vi "FrequencyShiftOneTarget_04012019.vi"(11 "Tones in":T3={"Config"={"UsrCfg"={"Paths"={"CfgFile"=path "", "LogFolder"=path "", "LogFile"=path "", "NAS path"=path "", "ThreshFile"=path "", "RedunFolder"=path ""}, "SampleRate"=0.0}, "FP_User"={"#NoiseSums"=1, "Max_df"=1, "AvgAvg"=FALSE, "#Avg"=0, "AutoCenter"=FALSE, "Inclin"={"Vmin"=0.0, "Vmax"=0.0, "Angle_min"=0.0, "Angle_max"=0.0, "Offset"=0.0, "Pos_Neg"=FALSE}, "1"={"Cal_"={"Fine"=0.0, "Coarse_"=0.0}, "Beac"={"Fine"=0.0, "Coarse_"=0.0}, "Scale"={"Step4"=0.0, "Step5"=0.0, "Step6"=0.0, "Step7"=0.0}, "Offset"=0.0, "Scale_Noise"=0.0, "Scale_Step1"=0.0, "Scale_In_RT"=0.0, "ScaleMeas"=0.0, "FreqsToRemove"=[], "Width"=[0, 1633], "ScaleMeasEnum"=enum."50", "FilterEnab"=enum."Step 1"}, "2"={"Cal_"={"Fine"=0.0, "Coarse_"=0.0}, "Beac"={"Fine"=0.0, "Coarse_"=0.0}, "Scale"={"Step4"=0.0, "Step5"=0.0, "Step6"=0.0, "Step7"=0.0}, "Offset"=0.0, "Scale_Noise"=0.0, "Scale_Step1"=0.0, "Scale_In_RT"=0.0, "ScaleMeas"=0.0, "FreqsToRemove"=[], "Width"=[0, 1633], "ScaleMeasEnum"=enum."50", "FilterEnab"=enum."Step 1"}, "3"={"Cal_"={"Fine"=0.0, "Coarse_"=0.0}, "Beac"={"Fine"=0.0, "Coarse_"=0.0}, "Scale"={"Step4"=0.0, "Step5"=0.0, "Step6"=0.0, "Step7"=0.0}, "Offset"=0.0, "Scale_Noise"=0.0, "Scale_Step1"=0.0, "Scale_In_RT"=0.0, "ScaleMeas"=0.0, "FreqsToRemove"=[], "Width"=[0, 1633], "ScaleMeasEnum"=enum."50", "FilterEnab"=enum."Step 1"}, "4"={"Cal_"={"Fine"=0.0, "Coarse_"=0.0}, "Beac"={"Fine"=0.0, "Coarse_"=0.0}, "Scale"={"Step4"=0.0, "Step5"=0.0, "Step6"=0.0, "Step7"=0.0}, "Offset"=0.0, "Scale_Noise"=0.0, "Scale_Step1"=0.0, "Scale_In_RT"=0.0, "ScaleMeas"=0.0, "FreqsToRemove"=[], "Width"=[0, 1633], "ScaleMeasEnum"=enum."50", "FilterEnab"=enum."Step 1"}, "Target to Probe"=enum."4", "SNR_Thresh"=1.0, "Paths"={"CfgFile"=path "", "LogFolder"=path "", "LogFile"=path "", "NAS path"=path "", "ThreshFile"=path "", "RedunFolder"=path ""}, "Connex_Location"="", "SimulateFPGA"=FALSE, "Deadband"=0.0}}, "FPGA"={"Target"=enum."4", "Channel"=enum."4", "Ref1"=refnum, "Ref2"=refnum}, "Now"={"Target"=enum."4", "SampleRate"=0.0, "AvgFreq"=0.0, "72_Shift_"=-24999462.633451957, "84_Shift_"=-24999462.633451957, "1"={"Cal"={"Shift_"=0.0, "Peak_ToFPGA"=-24999462.633451957, "MaxValue"=0.0, "MaxIndex"=0, "Tone"={"PkLocTrak"=0.0, "PkLocDisp"=0.0, "df_"=0.0, "ZoomPwr"=[], "Phase"=0.0, "PhaseOld"=0.0, "AboveThresh?"=FALSE, "MaxI"=0.0, "MaxQ"=0.0, "median"=0.0, "ISpect"=[], "QSpect"=[], "DeltaPhase"=0.0}, "TimeDomainI"=array[12500 elements], "TimeDomainQ"=array[12500 elements], "PwrSpectrum"=[], "RunningAvgFreq"=0.0, "ISpectPos"=[], "ISpectNeg"=[], "QSpectPos"=[], "QSpectNeg"=[], "10Hz_PwrSpectr"=[], "SNR"=0.0, "AliasWarn"=FALSE, "10Hz_Peak"=[], "ISpect+-"=[], "QSpect+-"=[], "TimeStamp"=timestamp(0 s since 1904-01-01), "I_Index"=array[12500 elements], "Q_Index"=array[12500 elements], "10MHz"=FALSE}, "Beac"={"Shift_"=0.0, "Peak_ToFPGA"=-24999462.633451957, "MaxValue"=0.0, "MaxIndex"=0, "Tone"={"PkLocTrak"=0.0, "PkLocDisp"=0.0, "df_"=0.0, "ZoomPwr"=[], "Phase"=0.0, "PhaseOld"=0.0, "AboveThresh?"=FALSE, "MaxI"=0.0, "MaxQ"=0.0, "median"=0.0, "ISpect"=[], "QSpect"=[], "DeltaPhase"=0.0}, "TimeDomainI"=array[12500 elements], "TimeDomainQ"=array[12500 elements], "PwrSpectrum"=[], "RunningAvgFreq"=0.0, "ISpectPos"=[], "ISpectNeg"=[], "QSpectPos"=[], "QSpectNeg"=[], "10Hz_PwrSpectr"=[], "SNR"=0.0, "AliasWarn"=FALSE, "10Hz_Peak"=[], "ISpect+-"=[], "QSpect+-"=[], "TimeStamp"=timestamp(0 s since 1904-01-01), "I_Index"=array[12500 elements], "Q_Index"=array[12500 elements], "10MHz"=FALSE}, "Time"=[], "Saturat"={"MeasMean0"=0.0, "MeasMean1"=0.0, "MeasMax"=0.0, "1_Max"=0.0, "4_Max"=0.0, "5_Max"=0.0, "6_Max"=0.0, "7_Max"=0.0}}, "2"={"Cal"={"Shift_"=0.0, "Peak_ToFPGA"=-24999462.633451957, "MaxValue"=0.0, "MaxIndex"=0, "Tone"={"PkLocTrak"=0.0, "PkLocDisp"=0.0, "df_"=0.0, "ZoomPwr"=[], "Phase"=0.0, "PhaseOld"=0.0, "AboveThresh?"=FALSE, "MaxI"=0.0, "MaxQ"=0.0, "median"=0.0, "ISpect"=[], "QSpect"=[], "DeltaPhase"=0.0}, "TimeDomainI"=array[12500 elements], "TimeDomainQ"=array[12500 elements], "PwrSpectrum"=[], "RunningAvgFreq"=0.0, "ISpectPos"=[], "ISpectNeg"=[], "QSpectPos"=[], "QSpectNeg"=[], "10Hz_PwrSpectr"=[], "SNR"=0.0, "AliasWarn"=FALSE, "10Hz_Peak"=[], "ISpect+-"=[], "QSpect+-"=[], "TimeStamp"=timestamp(0 s since 1904-01-01), "I_Index"=array[12500 elements], "Q_Index"=array[12500 elements], "10MHz"=FALSE}, "Beac"={"Shift_"=0.0, "Peak_ToFPGA"=-24999462.633451957, "MaxValue"=0.0, "MaxIndex"=0, "Tone"={"PkLocTrak"=0.0, "PkLocDisp"=0.0, "df_"=0.0, "ZoomPwr"=[], "Phase"=0.0, "PhaseOld"=0.0, "AboveThresh?"=FALSE, "MaxI"=0.0, "MaxQ"=0.0, "median"=0.0, "ISpect"=[], "QSpect"=[], "DeltaPhase"=0.0}, "TimeDomainI"=array[12500 elements], "TimeDomainQ"=array[12500 elements], "PwrSpectrum"=[], "RunningAvgFreq"=0.0, "ISpectPos"=[], "ISpectNeg"=[], "QSpectPos"=[], "QSpectNeg"=[], "10Hz_PwrSpectr"=[], "SNR"=0.0, "AliasWarn"=FALSE, "10Hz_Peak"=[], "ISpect+-"=[], "QSpect+-"=[], "TimeStamp"=timestamp(0 s since 1904-01-01), "I_Index"=array[12500 elements], "Q_Index"=array[12500 elements], "10MHz"=FALSE}, "Time"=[], "Saturat"={"MeasMean0"=0.0, "MeasMean1"=0.0, "MeasMax"=0.0, "1_Max"=0.0, "4_Max"=0.0, "5_Max"=0.0, "6_Max"=0.0, "7_Max"=0.0}}, "3"={"Cal"={"Shift_"=0.0, "Peak_ToFPGA"=-24999462.633451957, "MaxValue"=0.0, "MaxIndex"=0, "Tone"={"PkLocTrak"=0.0, "PkLocDisp"=0.0, "df_"=0.0, "ZoomPwr"=[], "Phase"=0.0, "PhaseOld"=0.0, "AboveThresh?"=FALSE, "MaxI"=0.0, "MaxQ"=0.0, "median"=0.0, "ISpect"=[], "QSpect"=[], "DeltaPhase"=0.0}, "TimeDomainI"=array[12500 elements], "TimeDomainQ"=array[12500 elements], "PwrSpectrum"=[], "RunningAvgFreq"=0.0, "ISpectPos"=[], "ISpectNeg"=[], "QSpectPos"=[], "QSpectNeg"=[], "10Hz_PwrSpectr"=[], "SNR"=0.0, "AliasWarn"=FALSE, "10Hz_Peak"=[], "ISpect+-"=[], "QSpect+-"=[], "TimeStamp"=timestamp(0 s since 1904-01-01), "I_Index"=array[12500 elements], "Q_Index"=array[12500 elements], "10MHz"=FALSE}, "Beac"={"Shift_"=0.0, "Peak_ToFPGA"=-24999462.633451957, "MaxValue"=0.0, "MaxIndex"=0, "Tone"={"PkLocTrak"=0.0, "PkLocDisp"=0.0, "df_"=0.0, "ZoomPwr"=[], "Phase"=0.0, "PhaseOld"=0.0, "AboveThresh?"=FALSE, "MaxI"=0.0, "MaxQ"=0.0, "median"=0.0, "ISpect"=[], "QSpect"=[], "DeltaPhase"=0.0}, "TimeDomainI"=array[12500 elements], "TimeDomainQ"=array[12500 elements], "PwrSpectrum"=[], "RunningAvgFreq"=0.0, "ISpectPos"=[], "ISpectNeg"=[], "QSpectPos"=[], "QSpectNeg"=[], "10Hz_PwrSpectr"=[], "SNR"=0.0, "AliasWarn"=FALSE, "10Hz_Peak"=[], "ISpect+-"=[], "QSpect+-"=[], "TimeStamp"=timestamp(0 s since 1904-01-01), "I_Index"=array[12500 elements], "Q_Index"=array[12500 elements], "10MHz"=FALSE}, "Time"=[], "Saturat"={"MeasMean0"=0.0, "MeasMean1"=0.0, "MeasMax"=0.0, "1_Max"=0.0, "4_Max"=0.0, "5_Max"=0.0, "6_Max"=0.0, "7_Max"=0.0}}, "4"={"Cal"={"Shift_"=0.0, "Peak_ToFPGA"=-24999462.633451957, "MaxValue"=0.0, "MaxIndex"=0, "Tone"={"PkLocTrak"=0.0, "PkLocDisp"=0.0, "df_"=0.0, "ZoomPwr"=[], "Phase"=0.0, "PhaseOld"=0.0, "AboveThresh?"=FALSE, "MaxI"=0.0, "MaxQ"=0.0, "median"=0.0, "ISpect"=[], "QSpect"=[], "DeltaPhase"=0.0}, "TimeDomainI"=array[12500 elements], "TimeDomainQ"=array[12500 elements], "PwrSpectrum"=[], "RunningAvgFreq"=0.0, "ISpectPos"=[], "ISpectNeg"=[], "QSpectPos"=[], "QSpectNeg"=[], "10Hz_PwrSpectr"=[], "SNR"=0.0, "AliasWarn"=FALSE, "10Hz_Peak"=[], "ISpect+-"=[], "QSpect+-"=[], "TimeStamp"=timestamp(0 s since 1904-01-01), "I_Index"=array[12500 elements], "Q_Index"=array[12500 elements], "10MHz"=FALSE}, "Beac"={"Shift_"=0.0, "Peak_ToFPGA"=-24999462.633451957, "MaxValue"=0.0, "MaxIndex"=0, "Tone"={"PkLocTrak"=0.0, "PkLocDisp"=0.0, "df_"=0.0, "ZoomPwr"=[], "Phase"=0.0, "PhaseOld"=0.0, "AboveThresh?"=FALSE, "MaxI"=0.0, "MaxQ"=0.0, "median"=0.0, "ISpect"=[], "QSpect"=[], "DeltaPhase"=0.0}, "TimeDomainI"=array[12500 elements], "TimeDomainQ"=array[12500 elements], "PwrSpectrum"=[], "RunningAvgFreq"=0.0, "ISpectPos"=[], "ISpectNeg"=[], "QSpectPos"=[], "QSpectNeg"=[], "10Hz_PwrSpectr"=[], "SNR"=0.0, "AliasWarn"=FALSE, "10Hz_Peak"=[], "ISpect+-"=[], "QSpect+-"=[], "TimeStamp"=timestamp(0 s since 1904-01-01), "I_Index"=array[12500 elements], "Q_Index"=array[12500 elements], "10MHz"=FALSE}, "Time"=[], "Saturat"={"MeasMean0"=0.0, "MeasMean1"=0.0, "MeasMax"=0.0, "1_Max"=0.0, "4_Max"=0.0, "5_Max"=0.0, "6_Max"=0.0, "7_Max"=0.0}}}, "FreqFiles"={"72"=path "", "84"=path ""}} {"Now"."4"."Beac"."Tone"."median" format="%0.2f"; "Now"."4"."Beac"."Tone"."MaxQ" format="%0.2f"; "Now"."4"."Cal"."Tone"."median" format="%0.2f"; "Now"."4"."Cal"."Tone"."MaxQ" format="%0.2f"; "Now"."3"."Beac"."Tone"."median" format="%0.2f"; "Now"."3"."Beac"."Tone"."MaxQ" format="%0.2f"; "Now"."3"."Cal"."Tone"."median" format="%0.2f"; "Now"."3"."Cal"."Tone"."MaxQ" format="%0.2f"; "Now"."2"."Beac"."Tone"."median" format="%0.2f"; "Now"."2"."Beac"."Tone"."MaxQ" format="%0.2f"; "Now"."2"."Cal"."Tone"."median" format="%0.2f"; "Now"."2"."Cal"."Tone"."MaxQ" format="%0.2f"; "Now"."1"."Beac"."Tone"."median" format="%0.2f"; "Now"."1"."Beac"."Tone"."MaxQ" format="%0.2f"; "Now"."1"."Cal"."Tone"."median" format="%0.2f"; "Now"."1"."Cal"."Tone"."MaxQ" format="%0.2f"; "Config"."FP_User"."Deadband" format="%#.0f"}) -> (3 "Tones out":T3={"Config"={"UsrCfg"={"Paths"={"CfgFile"=path "", "LogFolder"=path "", "LogFile"=path "", "NAS path"=path "", "ThreshFile"=path "", "RedunFolder"=path ""}, "SampleRate"=0.0}, "FP_User"={"#NoiseSums"=1, "Max_df"=1, "AvgAvg"=FALSE, "#Avg"=0, "AutoCenter"=FALSE, "Inclin"={"Vmin"=0.0, "Vmax"=0.0, "Angle_min"=0.0, "Angle_max"=0.0, "Offset"=0.0, "Pos_Neg"=FALSE}, "1"={"Cal_"={"Fine"=0.0, "Coarse_"=0.0}, "Beac"={"Fine"=0.0, "Coarse_"=0.0}, "Scale"={"Step4"=0.0, "Step5"=0.0, "Step6"=0.0, "Step7"=0.0}, "Offset"=0.0, "Scale_Noise"=0.0, "Scale_Step1"=0.0, "Scale_In_RT"=0.0, "ScaleMeas"=0.0, "FreqsToRemove"=[], "Width"=[0, 1633], "ScaleMeasEnum"=enum."50", "FilterEnab"=enum."Step 1"}, "2"={"Cal_"={"Fine"=0.0, "Coarse_"=0.0}, "Beac"={"Fine"=0.0, "Coarse_"=0.0}, "Scale"={"Step4"=0.0, "Step5"=0.0, "Step6"=0.0, "Step7"=0.0}, "Offset"=0.0, "Scale_Noise"=0.0, "Scale_Step1"=0.0, "Scale_In_RT"=0.0, "ScaleMeas"=0.0, "FreqsToRemove"=[], "Width"=[0, 1633], "ScaleMeasEnum"=enum."50", "FilterEnab"=enum."Step 1"}, "3"={"Cal_"={"Fine"=0.0, "Coarse_"=0.0}, "Beac"={"Fine"=0.0, "Coarse_"=0.0}, "Scale"={"Step4"=0.0, "Step5"=0.0, "Step6"=0.0, "Step7"=0.0}, "Offset"=0.0, "Scale_Noise"=0.0, "Scale_Step1"=0.0, "Scale_In_RT"=0.0, "ScaleMeas"=0.0, "FreqsToRemove"=[], "Width"=[0, 1633], "ScaleMeasEnum"=enum."50", "FilterEnab"=enum."Step 1"}, "4"={"Cal_"={"Fine"=0.0, "Coarse_"=0.0}, "Beac"={"Fine"=0.0, "Coarse_"=0.0}, "Scale"={"Step4"=0.0, "Step5"=0.0, "Step6"=0.0, "Step7"=0.0}, "Offset"=0.0, "Scale_Noise"=0.0, "Scale_Step1"=0.0, "Scale_In_RT"=0.0, "ScaleMeas"=0.0, "FreqsToRemove"=[], "Width"=[0, 1633], "ScaleMeasEnum"=enum."50", "FilterEnab"=enum."Step 1"}, "Target to Probe"=enum."4", "SNR_Thresh"=1.0, "Paths"={"CfgFile"=path "", "LogFolder"=path "", "LogFile"=path "", "NAS path"=path "", "ThreshFile"=path "", "RedunFolder"=path ""}, "Connex_Location"="", "SimulateFPGA"=FALSE, "Deadband"=0.0}}, "FPGA"={"Target"=enum."4", "Channel"=enum."4", "Ref1"=refnum, "Ref2"=refnum}, "Now"={"Target"=enum."4", "SampleRate"=0.0, "AvgFreq"=0.0, "72_Shift_"=-24999462.633451957, "84_Shift_"=-24999462.633451957, "1"={"Cal"={"Shift_"=0.0, "Peak_ToFPGA"=-24999462.633451957, "MaxValue"=0.0, "MaxIndex"=0, "Tone"={"PkLocTrak"=0.0, "PkLocDisp"=0.0, "df_"=0.0, "ZoomPwr"=[], "Phase"=0.0, "PhaseOld"=0.0, "AboveThresh?"=FALSE, "MaxI"=0.0, "MaxQ"=0.0, "median"=0.0, "ISpect"=[], "QSpect"=[], "DeltaPhase"=0.0}, "TimeDomainI"=array[12500 elements], "TimeDomainQ"=array[12500 elements], "PwrSpectrum"=[], "RunningAvgFreq"=0.0, "ISpectPos"=[], "ISpectNeg"=[], "QSpectPos"=[], "QSpectNeg"=[], "10Hz_PwrSpectr"=[], "SNR"=0.0, "AliasWarn"=FALSE, "10Hz_Peak"=[], "ISpect+-"=[], "QSpect+-"=[], "TimeStamp"=timestamp(0 s since 1904-01-01), "I_Index"=array[12500 elements], "Q_Index"=array[12500 elements], "10MHz"=FALSE}, "Beac"={"Shift_"=0.0, "Peak_ToFPGA"=-24999462.633451957, "MaxValue"=0.0, "MaxIndex"=0, "Tone"={"PkLocTrak"=0.0, "PkLocDisp"=0.0, "df_"=0.0, "ZoomPwr"=[], "Phase"=0.0, "PhaseOld"=0.0, "AboveThresh?"=FALSE, "MaxI"=0.0, "MaxQ"=0.0, "median"=0.0, "ISpect"=[], "QSpect"=[], "DeltaPhase"=0.0}, "TimeDomainI"=array[12500 elements], "TimeDomainQ"=array[12500 elements], "PwrSpectrum"=[], "RunningAvgFreq"=0.0, "ISpectPos"=[], "ISpectNeg"=[], "QSpectPos"=[], "QSpectNeg"=[], "10Hz_PwrSpectr"=[], "SNR"=0.0, "AliasWarn"=FALSE, "10Hz_Peak"=[], "ISpect+-"=[], "QSpect+-"=[], "TimeStamp"=timestamp(0 s since 1904-01-01), "I_Index"=array[12500 elements], "Q_Index"=array[12500 elements], "10MHz"=FALSE}, "Time"=[], "Saturat"={"MeasMean0"=0.0, "MeasMean1"=0.0, "MeasMax"=0.0, "1_Max"=0.0, "4_Max"=0.0, "5_Max"=0.0, "6_Max"=0.0, "7_Max"=0.0}}, "2"={"Cal"={"Shift_"=0.0, "Peak_ToFPGA"=-24999462.633451957, "MaxValue"=0.0, "MaxIndex"=0, "Tone"={"PkLocTrak"=0.0, "PkLocDisp"=0.0, "df_"=0.0, "ZoomPwr"=[], "Phase"=0.0, "PhaseOld"=0.0, "AboveThresh?"=FALSE, "MaxI"=0.0, "MaxQ"=0.0, "median"=0.0, "ISpect"=[], "QSpect"=[], "DeltaPhase"=0.0}, "TimeDomainI"=array[12500 elements], "TimeDomainQ"=array[12500 elements], "PwrSpectrum"=[], "RunningAvgFreq"=0.0, "ISpectPos"=[], "ISpectNeg"=[], "QSpectPos"=[], "QSpectNeg"=[], "10Hz_PwrSpectr"=[], "SNR"=0.0, "AliasWarn"=FALSE, "10Hz_Peak"=[], "ISpect+-"=[], "QSpect+-"=[], "TimeStamp"=timestamp(0 s since 1904-01-01), "I_Index"=array[12500 elements], "Q_Index"=array[12500 elements], "10MHz"=FALSE}, "Beac"={"Shift_"=0.0, "Peak_ToFPGA"=-24999462.633451957, "MaxValue"=0.0, "MaxIndex"=0, "Tone"={"PkLocTrak"=0.0, "PkLocDisp"=0.0, "df_"=0.0, "ZoomPwr"=[], "Phase"=0.0, "PhaseOld"=0.0, "AboveThresh?"=FALSE, "MaxI"=0.0, "MaxQ"=0.0, "median"=0.0, "ISpect"=[], "QSpect"=[], "DeltaPhase"=0.0}, "TimeDomainI"=array[12500 elements], "TimeDomainQ"=array[12500 elements], "PwrSpectrum"=[], "RunningAvgFreq"=0.0, "ISpectPos"=[], "ISpectNeg"=[], "QSpectPos"=[], "QSpectNeg"=[], "10Hz_PwrSpectr"=[], "SNR"=0.0, "AliasWarn"=FALSE, "10Hz_Peak"=[], "ISpect+-"=[], "QSpect+-"=[], "TimeStamp"=timestamp(0 s since 1904-01-01), "I_Index"=array[12500 elements], "Q_Index"=array[12500 elements], "10MHz"=FALSE}, "Time"=[], "Saturat"={"MeasMean0"=0.0, "MeasMean1"=0.0, "MeasMax"=0.0, "1_Max"=0.0, "4_Max"=0.0, "5_Max"=0.0, "6_Max"=0.0, "7_Max"=0.0}}, "3"={"Cal"={"Shift_"=0.0, "Peak_ToFPGA"=-24999462.633451957, "MaxValue"=0.0, "MaxIndex"=0, "Tone"={"PkLocTrak"=0.0, "PkLocDisp"=0.0, "df_"=0.0, "ZoomPwr"=[], "Phase"=0.0, "PhaseOld"=0.0, "AboveThresh?"=FALSE, "MaxI"=0.0, "MaxQ"=0.0, "median"=0.0, "ISpect"=[], "QSpect"=[], "DeltaPhase"=0.0}, "TimeDomainI"=array[12500 elements], "TimeDomainQ"=array[12500 elements], "PwrSpectrum"=[], "RunningAvgFreq"=0.0, "ISpectPos"=[], "ISpectNeg"=[], "QSpectPos"=[], "QSpectNeg"=[], "10Hz_PwrSpectr"=[], "SNR"=0.0, "AliasWarn"=FALSE, "10Hz_Peak"=[], "ISpect+-"=[], "QSpect+-"=[], "TimeStamp"=timestamp(0 s since 1904-01-01), "I_Index"=array[12500 elements], "Q_Index"=array[12500 elements], "10MHz"=FALSE}, "Beac"={"Shift_"=0.0, "Peak_ToFPGA"=-24999462.633451957, "MaxValue"=0.0, "MaxIndex"=0, "Tone"={"PkLocTrak"=0.0, "PkLocDisp"=0.0, "df_"=0.0, "ZoomPwr"=[], "Phase"=0.0, "PhaseOld"=0.0, "AboveThresh?"=FALSE, "MaxI"=0.0, "MaxQ"=0.0, "median"=0.0, "ISpect"=[], "QSpect"=[], "DeltaPhase"=0.0}, "TimeDomainI"=array[12500 elements], "TimeDomainQ"=array[12500 elements], "PwrSpectrum"=[], "RunningAvgFreq"=0.0, "ISpectPos"=[], "ISpectNeg"=[], "QSpectPos"=[], "QSpectNeg"=[], "10Hz_PwrSpectr"=[], "SNR"=0.0, "AliasWarn"=FALSE, "10Hz_Peak"=[], "ISpect+-"=[], "QSpect+-"=[], "TimeStamp"=timestamp(0 s since 1904-01-01), "I_Index"=array[12500 elements], "Q_Index"=array[12500 elements], "10MHz"=FALSE}, "Time"=[], "Saturat"={"MeasMean0"=0.0, "MeasMean1"=0.0, "MeasMax"=0.0, "1_Max"=0.0, "4_Max"=0.0, "5_Max"=0.0, "6_Max"=0.0, "7_Max"=0.0}}, "4"={"Cal"={"Shift_"=0.0, "Peak_ToFPGA"=-24999462.633451957, "MaxValue"=0.0, "MaxIndex"=0, "Tone"={"PkLocTrak"=0.0, "PkLocDisp"=0.0, "df_"=0.0, "ZoomPwr"=[], "Phase"=0.0, "PhaseOld"=0.0, "AboveThresh?"=FALSE, "MaxI"=0.0, "MaxQ"=0.0, "median"=0.0, "ISpect"=[], "QSpect"=[], "DeltaPhase"=0.0}, "TimeDomainI"=array[12500 elements], "TimeDomainQ"=array[12500 elements], "PwrSpectrum"=[], "RunningAvgFreq"=0.0, "ISpectPos"=[], "ISpectNeg"=[], "QSpectPos"=[], "QSpectNeg"=[], "10Hz_PwrSpectr"=[], "SNR"=0.0, "AliasWarn"=FALSE, "10Hz_Peak"=[], "ISpect+-"=[], "QSpect+-"=[], "TimeStamp"=timestamp(0 s since 1904-01-01), "I_Index"=array[12500 elements], "Q_Index"=array[12500 elements], "10MHz"=FALSE}, "Beac"={"Shift_"=0.0, "Peak_ToFPGA"=-24999462.633451957, "MaxValue"=0.0, "MaxIndex"=0, "Tone"={"PkLocTrak"=0.0, "PkLocDisp"=0.0, "df_"=0.0, "ZoomPwr"=[], "Phase"=0.0, "PhaseOld"=0.0, "AboveThresh?"=FALSE, "MaxI"=0.0, "MaxQ"=0.0, "median"=0.0, "ISpect"=[], "QSpect"=[], "DeltaPhase"=0.0}, "TimeDomainI"=array[12500 elements], "TimeDomainQ"=array[12500 elements], "PwrSpectrum"=[], "RunningAvgFreq"=0.0, "ISpectPos"=[], "ISpectNeg"=[], "QSpectPos"=[], "QSpectNeg"=[], "10Hz_PwrSpectr"=[], "SNR"=0.0, "AliasWarn"=FALSE, "10Hz_Peak"=[], "ISpect+-"=[], "QSpect+-"=[], "TimeStamp"=timestamp(0 s since 1904-01-01), "I_Index"=array[12500 elements], "Q_Index"=array[12500 elements], "10MHz"=FALSE}, "Time"=[], "Saturat"={"MeasMean0"=0.0, "MeasMean1"=0.0, "MeasMax"=0.0, "1_Max"=0.0, "4_Max"=0.0, "5_Max"=0.0, "6_Max"=0.0, "7_Max"=0.0}}}, "FreqFiles"={"72"=path "", "84"=path ""}} {"Now"."4"."Beac"."Tone"."median" format="%0.2f"; "Now"."4"."Beac"."Tone"."MaxQ" format="%0.2f"; "Now"."4"."Cal"."Tone"."median" format="%0.2f"; "Now"."4"."Cal"."Tone"."MaxQ" format="%0.2f"; "Now"."3"."Beac"."Tone"."median" format="%0.2f"; "Now"."3"."Beac"."Tone"."MaxQ" format="%0.2f"; "Now"."3"."Cal"."Tone"."median" format="%0.2f"; "Now"."3"."Cal"."Tone"."MaxQ" format="%0.2f"; "Now"."2"."Beac"."Tone"."median" format="%0.2f"; "Now"."2"."Beac"."Tone"."MaxQ" format="%0.2f"; "Now"."2"."Cal"."Tone"."median" format="%0.2f"; "Now"."2"."Cal"."Tone"."MaxQ" format="%0.2f"; "Now"."1"."Beac"."Tone"."median" format="%0.2f"; "Now"."1"."Beac"."Tone"."MaxQ" format="%0.2f"; "Now"."1"."Cal"."Tone"."median" format="%0.2f"; "Now"."1"."Cal"."Tone"."MaxQ" format="%0.2f"; "Config"."FP_User"."Deadband" format="%#.0f"})   [LabVIEW 2018]
uses:
  Controls/Clusts/Tones_Loop.ctl
  Controls/Clusts/Config_Clust.ctl
  Controls/Clusts/UserConfig.ctl
  Controls/PathsCluster.ctl
  Controls/Clusts/FrontPanel_UserConfig.ctl
  Controls/Clusts/Inclinometer_User_Cfg.ctl
  Controls/Clusts/FP_UserTargetConfig.ctl
  Controls/Clusts/FreqShift.ctl
  Controls/Clusts/FPGA_Scale.ctl
  Controls/Enums/ScaleMeasure.ctl
  Controls/RadioButtons/FilterEnableRadio.ctl
  Controls/Enums/TargetNumber.ctl
  Controls/Clusts/FPGA_Config_Clust.ctl
  Controls/Clusts/NowAllTones.ctl
  Controls/Clusts/TargetToneData.ctl
  Controls/Clusts/ChannelToneData.ctl
  Controls/ToneInfoClust.ctl
  Controls/Clusts/SaturationMonitor.ctl
  Controls/Clusts/FreqFilePaths.ctl
panel:
  in  "Cal":T1={"Shift_"=-24999462.633451957, "Peak_ToFPGA"=-24999462.633451957, "MaxValue"=0.0, "MaxIndex"=0, "Tone"={"PkLocTrak"=0.0, "PkLocDisp"=0.0, "df_"=0.0, "ZoomPwr"=[], "Phase"=0.0, "PhaseOld"=0.0, "AboveThresh?"=FALSE, "MaxI"=0.0, "MaxQ"=0.0, "median"=0.0, "ISpect"=[], "QSpect"=[], "DeltaPhase"=0.0}, "TimeDomainI"=array[12500 elements], "TimeDomainQ"=array[12500 elements], "PwrSpectrum"=[], "RunningAvgFreq"=0.0, "ISpectPos"=[], "ISpectNeg"=[], "QSpectPos"=[], "QSpectNeg"=[], "10Hz_PwrSpectr"=[], "SNR"=0.0, "AliasWarn"=FALSE, "10Hz_Peak"=[], "ISpect+-"=[], "QSpect+-"=[], "TimeStamp"=timestamp(0 s since 1904-01-01), "I_Index"=array[12500 elements], "Q_Index"=array[12500 elements], "10MHz"=FALSE} {"Tone"."median" format="%0.2f"; "Tone"."MaxQ" format="%0.2f"}
  in  "output cluster":T1={"Shift_"=-24999462.633451957, "Peak_ToFPGA"=-24999462.633451957, "MaxValue"=0.0, "MaxIndex"=0, "Tone"={"PkLocTrak"=0.0, "PkLocDisp"=0.0, "df_"=0.0, "ZoomPwr"=[], "Phase"=0.0, "PhaseOld"=0.0, "AboveThresh?"=FALSE, "MaxI"=0.0, "MaxQ"=0.0, "median"=0.0, "ISpect"=[], "QSpect"=[], "DeltaPhase"=0.0}, "TimeDomainI"=array[12500 elements], "TimeDomainQ"=array[12500 elements], "PwrSpectrum"=[], "RunningAvgFreq"=0.0, "ISpectPos"=[], "ISpectNeg"=[], "QSpectPos"=[], "QSpectNeg"=[], "10Hz_PwrSpectr"=[], "SNR"=0.0, "AliasWarn"=FALSE, "10Hz_Peak"=[], "ISpect+-"=[], "QSpect+-"=[], "TimeStamp"=timestamp(0 s since 1904-01-01), "I_Index"=array[12500 elements], "Q_Index"=array[12500 elements], "10MHz"=FALSE} {"Tone"."median" format="%0.2f"; "Tone"."MaxQ" format="%0.2f"}
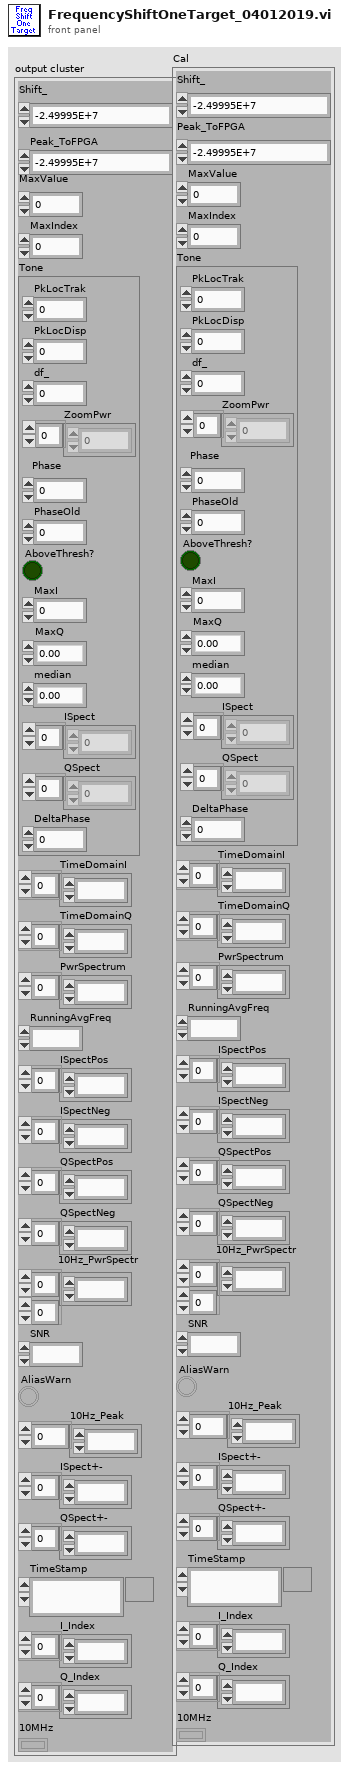
[diagram p1: front panel]
types:
  T1 = typedef "ChannelToneData.ctl" = cluster{"Shift_":dbl, "Peak_ToFPGA":dbl, "MaxValue":dbl, "MaxIndex":i32, "Tone":T2, "TimeDomainI":ext[], "TimeDomainQ":ext[], "PwrSpectrum":dbl[], "RunningAvgFreq":dbl, "ISpectPos":dbl[], "ISpectNeg":dbl[], "QSpectPos":dbl[], "QSpectNeg":dbl[], "10Hz_PwrSpectr":dbl[][], "SNR":dbl, "AliasWarn":bool, "10Hz_Peak":dbl[], "ISpect+-":dbl[], "QSpect+-":dbl[], "TimeStamp":timestamp, "I_Index":ext[], "Q_Index":ext[], "10MHz":bool}
  T2 = typedef "ToneInfoClust.ctl" = cluster{"PkLocTrak":dbl, "PkLocDisp":dbl, "df_":dbl, "ZoomPwr":dbl[], "Phase":dbl, "PhaseOld":dbl, "AboveThresh?":bool, "MaxI":dbl, "MaxQ":dbl, "median":dbl, "ISpect":dbl[], "QSpect":dbl[], "DeltaPhase":dbl}
  T3 = typedef "Tones_Loop.ctl" = cluster{"Config":T4, "FPGA":T15, "Now":T16, "FreqFiles":T19}
  T4 = typedef "Config_Clust.ctl" = cluster{"UsrCfg":T5, "FP_User":T7}
  T5 = typedef "UserConfig.ctl" = cluster{"Paths":T6, "SampleRate":dbl}
  T6 = typedef "PathsCluster.ctl" = cluster{"CfgFile":path, "LogFolder":path, "LogFile":path, "NAS path":path, "ThreshFile":path, "RedunFolder":path}
  T7 = typedef "FrontPanel_UserConfig.ctl" = cluster{"#NoiseSums":u32, "Max_df":u32, "AvgAvg":bool, "#Avg":u16, "AutoCenter":bool, "Inclin":T8, "1":T9, "2":T9, "3":T9, "4":T9, "Target to Probe":T14, "SNR_Thresh":dbl, "Paths":T6, "Connex_Location":string, "SimulateFPGA":bool, "Deadband":dbl}
  T8 = typedef "Inclinometer_User_Cfg.ctl" = cluster{"Vmin":dbl, "Vmax":dbl, "Angle_min":dbl, "Angle_max":dbl, "Offset":dbl, "Pos_Neg":bool}
  T9 = typedef "FP_UserTargetConfig.ctl" = cluster{"Cal_":T10, "Beac":T10, "Scale":T11, "Offset":fxp<+/-,16,16>, "Scale_Noise":fxp<+/-,30,30>, "Scale_Step1":fxp<+/-,17,17>, "Scale_In_RT":ext, "ScaleMeas":fxp<+/-,16,1>, "FreqsToRemove":i32[], "Width":i32[], "ScaleMeasEnum":T12, "FilterEnab":T13}
  T10 = typedef "FreqShift.ctl" = cluster{"Fine":dbl, "Coarse_":dbl}
  T11 = typedef "FPGA_Scale.ctl" = cluster{"Step4":fxp<+/-,23,23>, "Step5":fxp<+/-,23,23>, "Step6":fxp<+/-,23,23>, "Step7":fxp<+/-,23,23>}
  T12 = typedef "ScaleMeasure.ctl" = enum16{"1", "10", "50", "42"}
  T13 = typedef "FilterEnableRadio.ctl" = enum32{"None", "Step 1", "Frequency Shift", "Step 4", "Step 5", "Step 6", "Step 7"}
  T14 = typedef "TargetNumber.ctl" = enum16{"1", "2", "3", "4"}
  T15 = typedef "FPGA_Config_Clust.ctl" = cluster{"Target":T14, "Channel":T14, "Ref1":refnum<k20>, "Ref2":refnum<k20>}
  T16 = typedef "NowAllTones.ctl" = cluster{"Target":T14, "SampleRate":dbl, "AvgFreq":dbl, "72_Shift_":dbl, "84_Shift_":dbl, "1":T17, "2":T17, "3":T17, "4":T17}
  T17 = typedef "TargetToneData.ctl" = cluster{"Cal":T1, "Beac":T1, "Time":timestamp[], "Saturat":T18}
  T18 = typedef "SaturationMonitor.ctl" = cluster{"MeasMean0":dbl, "MeasMean1":dbl, "MeasMax":dbl, "1_Max":dbl, "4_Max":dbl, "5_Max":dbl, "6_Max":dbl, "7_Max":dbl}
  T19 = typedef "FreqFilePaths.ctl" = cluster{"72":path, "84":path}
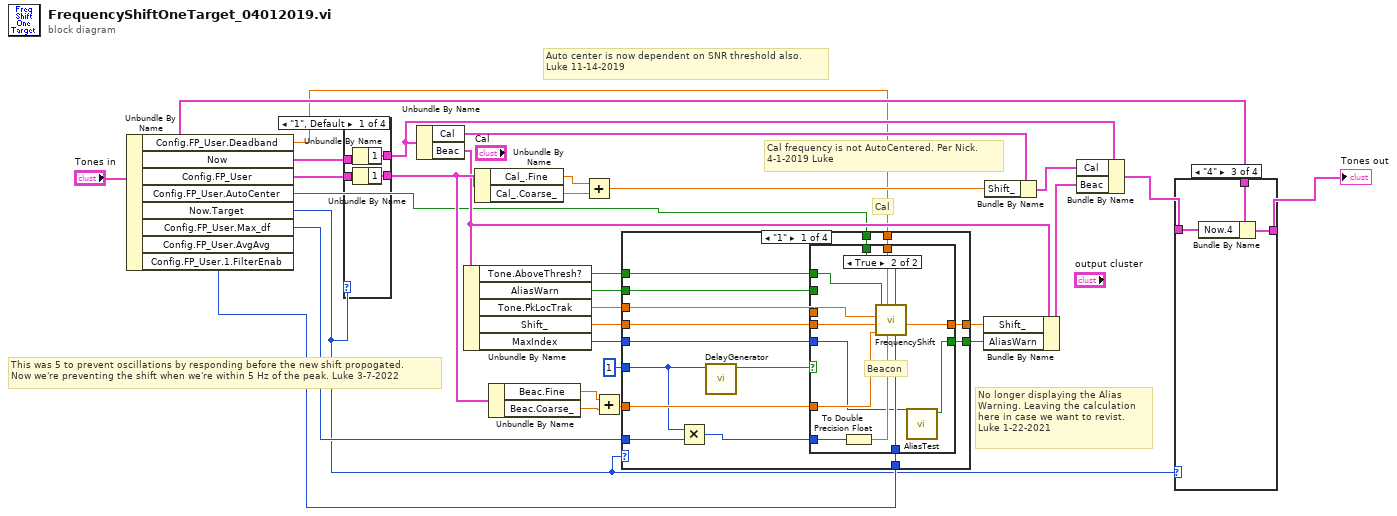
[diagram p0: block diagram]
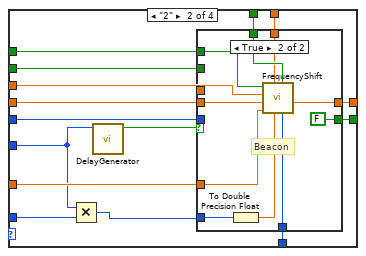
[diagram p3: hidden frame]
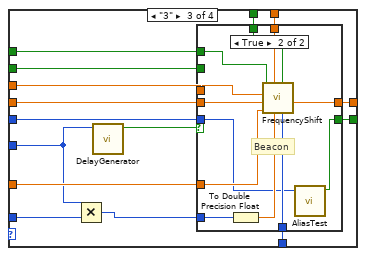
[diagram p5: hidden frame]
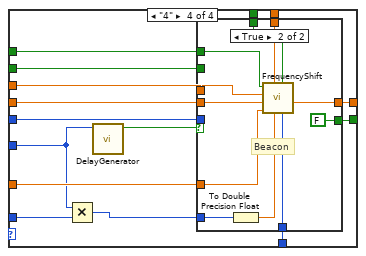
[diagram p7: hidden frame]
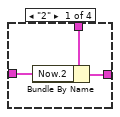
[diagram p9: hidden frame]
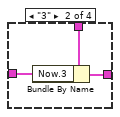
[diagram p10: hidden frame]
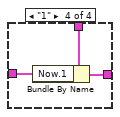
[diagram p11: hidden frame]
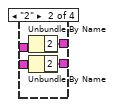
[diagram p12: hidden frame]
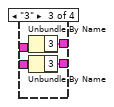
[diagram p13: hidden frame]
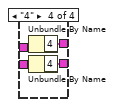
[diagram p14: hidden frame]
diagram:
  # "This was 5 to prevent oscillations by responding before the new shift propogated.\nNow we're preventing the shift when we're within 5 Hz of the peak. Luke 3-7-2022"
  # "No longer displaying the Alias\nWarning. Leaving the calculation\nhere in case we want to revist.\nLuke 1-22-2021"
  # "Auto center is now dependent on SNR threshold also.\nLuke 11-14-2019"
  # "Cal frequency is not AutoCentered. Per Nick.\n4-1-2019 Luke"
  # "Cal"
  n1 = Unbundle By Name("Tones in") -> ("Config.FP_User.Deadband"=w1:dbl, "Now"=w30:T16, "Config.FP_User"=w17:T7, "Config.FP_User.AutoCenter"=w3:bool, "Now.Target"=w7:T14, "Config.FP_User.Max_df"=w8:u32, "Config.FP_User.1.FilterEnab"=w10:T13)  [unwired: 1 out]
  n2 = case shown="\"1\", Default" w7 {
    tunnel: [w34 w38 w42 w46] -> w15
    tunnel: w17 -> [w33 w37 w41 w45]
    tunnel: [w32 w36 w40 w44] -> w28
    tunnel: w30 -> [w31 w35 w39 w43]
    frame "1", Default {
      n3 = Unbundle By Name(w31) -> ("1"=w34:T17)
      n4 = Unbundle By Name(w33) -> ("1"=w32:T9)
    }
    frame "2" {
      n5 = Unbundle By Name(w35) -> ("2"=w38:T17)
      n6 = Unbundle By Name(w37) -> ("2"=w36:T9)
    }
    frame "3" {
      n7 = Unbundle By Name(w39) -> ("3"=w42:T17)
      n8 = Unbundle By Name(w41) -> ("3"=w40:T9)
    }
    frame "4" {
      n9 = Unbundle By Name(w43) -> ("4"=w46:T17)
      n10 = Unbundle By Name(w45) -> ("4"=w44:T9)
    }
  }
  n11 = Unbundle By Name(w15) -> ("Cal"=w18:T1, "Beac"=w23:T1)
  n12 = Unbundle By Name(w23) -> ("Tone.AboveThresh?"=w2:bool, "AliasWarn"=w6:bool, "Tone.PkLocTrak"=w12:dbl, "Shift_"=w11:dbl, "MaxIndex"=w5:i32)
  n13 = Unbundle By Name(w28) -> ("Cal_.Fine"=w19:dbl, "Cal_.Coarse_"=w20:dbl)
  n14 = Unbundle By Name(w28) -> ("Beac.Fine"=w21:dbl, "Beac.Coarse_"=w22:dbl)
  n15 = Add(x=w19, y=w20) -> (x+y=w14:dbl)
  n16 = Add(x=w21, y=w22) -> (x+y=w13:dbl)
  n17 = case shown="\"1\"" w7 {
    tunnel: [w61 w90 w118 w147] -> w24
    tunnel: w3 -> [w60 w89 w117 w146]
    tunnel: w13 -> [w59 w88 w116 w145]
    tunnel: w12 -> [w58 w87 w115 w144]
    tunnel: w11 -> [w57 w86 w114 w143]
    tunnel: w10 -> [w56 w85 w113 w142]
    tunnel: u32 1 ("y") -> [w54 w82 w111 w140]
    tunnel: w8 -> [w52 w83 w109 w138]
    tunnel: [w51 w80 w108 w137] -> w4
    tunnel: w6 -> [w50 w79 w107 w136]
    tunnel: w5 -> [w49 w78 w106 w135]
    tunnel: w2 -> [w48 w77 w105 w134]
    tunnel: w1 -> [w47 w76 w104 w133]
    frame "1" {
      n18 = Multiply(x=w54, y=w52) -> (x*y=w53:u32)
      n19 = call "DelayGenerator.vi"("Delay(cycles)"=w54) -> ("Trigger"=w55:bool)  [unwired: 10 in]
      n20 = case shown="True" w55 {
        tunnel: [w63 w75] -> w61
        tunnel: w60 -> [_ w65]
        tunnel: w59 -> [_ w74]
        tunnel: w58 -> [_ w73]
        tunnel: w57 -> [w63 w71]
        tunnel: w56 -> [_ w70]
        tunnel: w53 -> [_ w69]
        tunnel: [w62 w67] -> w51
        tunnel: w50 -> [w62 _]
        tunnel: w49 -> [_ w68]
        tunnel: w48 -> [_ w66]
        tunnel: w47 -> [_ w64]
        frame False {
        }
        frame True {
          # "Beacon"
          n21 = To Double Precision Float(number=w69) -> (double precision float=w72:dbl)
          n22 = call "FrequencyShift.vi"("Radio Buttons"=w70, "AutoCenter"=w65, "delta f"=w72, "Deadband"=w64, "ManualShift"=w74, "Shift_"=w71, "NewestPeak"=w73, "Tone.AboveThresh?"=w66) -> ("TotalShift"=w75:dbl)  [unwired: 3 in]
          n23 = call "AliasTest.vi"("MaxIndex"=w68) -> ("Alias warning"=w67:bool)  [unwired: 10 in]
        }
      }
    }
    frame "2" {
      n24 = Multiply(x=w82, y=w83) -> (x*y=w81:u32)
      n25 = call "DelayGenerator.vi"("Delay(cycles)"=w82) -> ("Trigger"=w84:bool)  [unwired: 10 in]
      n26 = case shown="True" w84 {
        tunnel: [w92 w103] -> w90
        tunnel: w89 -> [_ w96]
        tunnel: w88 -> [_ w102]
        tunnel: w87 -> [_ w101]
        tunnel: w86 -> [w92 w99]
        tunnel: w85 -> [_ w98]
        tunnel: w81 -> [_ w97]
        tunnel: [w91 FALSE ("AliasWarn")] -> w80
        tunnel: w79 -> [w91 _]
        tunnel: w78 -> [_ _]
        tunnel: w77 -> [_ w95]
        tunnel: w76 -> [_ w93]
        frame False {
        }
        frame True {
          # "Beacon"
          n27 = To Double Precision Float(number=w97) -> (double precision float=w100:dbl)
          n28 = call "FrequencyShift.vi"("Radio Buttons"=w98, "AutoCenter"=w96, "delta f"=w100, "Deadband"=w93, "ManualShift"=w102, "Shift_"=w99, "NewestPeak"=w101, "Tone.AboveThresh?"=w95) -> ("TotalShift"=w103:dbl)  [unwired: 3 in]
        }
      }
    }
    frame "3" {
      n29 = Multiply(x=w111, y=w109) -> (x*y=w110:u32)
      n30 = call "DelayGenerator.vi"("Delay(cycles)"=w111) -> ("Trigger"=w112:bool)  [unwired: 10 in]
      n31 = case shown="True" w112 {
        tunnel: [w120 w132] -> w118
        tunnel: w117 -> [_ w123]
        tunnel: w116 -> [_ w131]
        tunnel: w115 -> [_ w130]
        tunnel: w114 -> [w120 w128]
        tunnel: w113 -> [_ w127]
        tunnel: w110 -> [_ w126]
        tunnel: [w119 w124] -> w108
        tunnel: w107 -> [w119 _]
        tunnel: w106 -> [_ w125]
        tunnel: w105 -> [_ w122]
        tunnel: w104 -> [_ w121]
        frame False {
        }
        frame True {
          # "Beacon"
          n32 = To Double Precision Float(number=w126) -> (double precision float=w129:dbl)
          n33 = call "FrequencyShift.vi"("Radio Buttons"=w127, "AutoCenter"=w123, "delta f"=w129, "Deadband"=w121, "ManualShift"=w131, "Shift_"=w128, "NewestPeak"=w130, "Tone.AboveThresh?"=w122) -> ("TotalShift"=w132:dbl)  [unwired: 3 in]
          n34 = call "AliasTest.vi"("MaxIndex"=w125) -> ("Alias warning"=w124:bool)  [unwired: 10 in]
        }
      }
    }
    frame "4" {
      n35 = Multiply(x=w140, y=w138) -> (x*y=w139:u32)
      n36 = call "DelayGenerator.vi"("Delay(cycles)"=w140) -> ("Trigger"=w141:bool)  [unwired: 10 in]
      n37 = case shown="True" w141 {
        tunnel: [w149 w160] -> w147
        tunnel: w146 -> [_ w153]
        tunnel: w145 -> [_ w159]
        tunnel: w144 -> [_ w158]
        tunnel: w143 -> [w149 w156]
        tunnel: w142 -> [_ w155]
        tunnel: w139 -> [_ w154]
        tunnel: [w148 FALSE ("AliasWarn")] -> w137
        tunnel: w136 -> [w148 _]
        tunnel: w135 -> [_ _]
        tunnel: w134 -> [_ w152]
        tunnel: w133 -> [_ w150]
        frame False {
        }
        frame True {
          # "Beacon"
          n38 = To Double Precision Float(number=w154) -> (double precision float=w157:dbl)
          n39 = call "FrequencyShift.vi"("Radio Buttons"=w155, "AutoCenter"=w153, "delta f"=w157, "Deadband"=w150, "ManualShift"=w159, "Shift_"=w156, "NewestPeak"=w158, "Tone.AboveThresh?"=w152) -> ("TotalShift"=w160:dbl)  [unwired: 3 in]
        }
      }
    }
  }
  n40 = Bundle By Name(cluster=w23, "Shift_"=w24, "AliasWarn"=w4) -> (w25:T1)
  n41 = Bundle By Name(cluster=w18, "Shift_"=w14) -> (w16:T1)
  n42 = Bundle By Name(cluster=w15, "Cal"=w16, "Beac"=w25) -> (w26:T17)
  n43 = case shown="\"4\"" w7 {
    tunnel: w26 -> [w163 w166 w169 w172]
    tunnel: "Tones in" -> [w162 w165 w168 w171]
    tunnel: [w161 w164 w167 w170] -> w29
    frame "2" {
      n44 = Bundle By Name(cluster=w162, "Now.2"=w163) -> (w161:T3)
    }
    frame "3" {
      n45 = Bundle By Name(cluster=w165, "Now.3"=w166) -> (w164:T3)
    }
    frame "4" {
      n46 = Bundle By Name(cluster=w168, "Now.4"=w169) -> (w167:T3)
    }
    frame "1" {
      n47 = Bundle By Name(cluster=w171, "Now.1"=w172) -> (w170:T3)
    }
  }
  "Tones out" <- w29
